vi "Home.vi"(8 "error in (no error)":errorcluster, 10 "Axis":i32=1, 11 "VISA resource name in":refnum<visa-resource-name>) -> (0 "error out":errorcluster, 3 "VISA resource name out":refnum<visa-resource-name>)   [LabVIEW 2015]
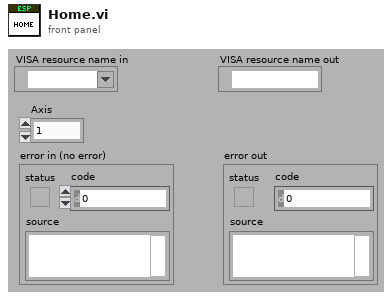
[diagram p1: front panel]
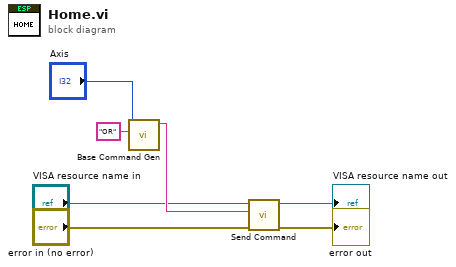
[diagram p0: block diagram]
diagram:
  n1 = call "Base Command Gen.vi"("Command"="OR", "xx"="Axis") -> ("Command"=w4:string)  [unwired: 9 in]
  n2 = call "Send Command.vi"("error out (no error)"="error in (no error)", "Command"=w4, "VISA resource name in"="VISA resource name in") -> ("error out"=→"error out":errorcluster, "VISA resource name out"=→"VISA resource name out":refnum<visa-resource-name>)  [unwired: 7 in]
